vi "Get Decimal Places.vi"(8 "error in (no error)":errorcluster, 10 "Channel":T2, 11 "EPU452 in":refnum<class "EPU452.lvclass">) -> (0 "error out":errorcluster, 1 "No. of Decimal Places":T1=enum."auto", 2 "Response":string, 3 "EPU452 out":refnum<class "EPU452.lvclass">)   [LabVIEW 2018, in "EPU452.lvclass"]
uses:
  EPU452.lvclass
  Controls/Channels.ctl
  Controls/Decimal Places.ctl
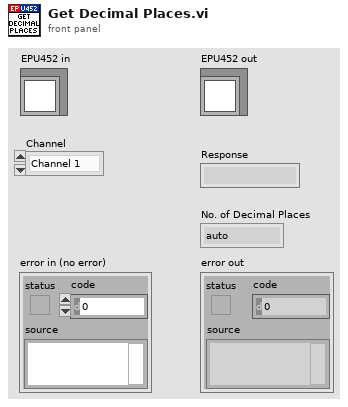
[diagram p1: front panel]
types:
  T1 = typedef "EPU452.lvclass/Decimal Places.ctl" = enum16{"0", "1", "2", "3", "4", "5", "6", "auto"}
  T2 = typedef "EPU452.lvclass/Channels.ctl" = enum16{"Channel 1", "Channel 2", "Channel 3", "Channel 4"}
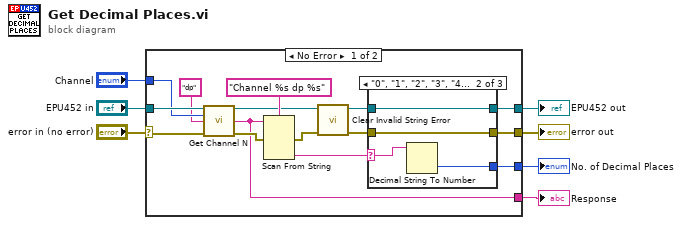
[diagram p0: block diagram]
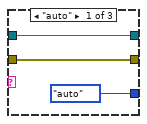
[diagram p2: hidden frame]
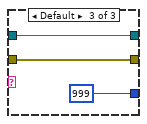
[diagram p3: hidden frame]
diagram:
  n1 = case shown="No Error" "error in (no error)" {
    selector: "error in (no error)" -> [w19 w34]
    tunnel: [w11 w34] -> w6
    tunnel: [w12 w33] -> w4
    tunnel: "EPU452 in" -> [w22 w33]
    tunnel: "Channel" -> [w21 _]
    tunnel: [w10 _] -> w2
    tunnel: [w9 _] -> w1
    frame No Error {
      n2 = call "Get Channel N.vi"("EPU452 in"=w22, "Channel"=w21, "Function"="dp", "error in (no error)"=w19) -> ("EPU452 out"=w16:refnum<class "EPU452.lvclass">, "Response"=w9:string, "error out"=w17:errorcluster)  [unwired: 9 in]
      n3 = Scan From String(format string="Channel %s dp %s" ("Function"), input string=w9, error in=w17) -> (error out=w15:errorcluster, output 2=w8:string)  [unwired: 4 in, 2 out]
      n4 = call "Clear Invalid String Error.vi"("error in (no error)"=w15, "EPU452 in"=w16) -> ("error out"=w14:errorcluster, "EPU452 out"=w13:refnum<class "EPU452.lvclass">)  [unwired: 8 in]
      n5 = case shown="\"0\", \"1\", \"2\", \"3\", \"4\", \"5\", \"6\"" w8 {
        selector: w8 -> [_ w29 _]
        tunnel: w14 -> [w24 w27 w30]
        tunnel: w13 -> [w23 w26 w31]
        tunnel: [Decimal_Places."auto" ("No. of Decimal Places") w28 999] -> w10
        tunnel: [w24 w27 w30] -> w11
        tunnel: [w23 w26 w31] -> w12
        frame "auto" {
        }
        frame "0", "1", "2", "3", "4", "5", "6" {
          n6 = Decimal String To Number(string=w29) -> (number=w28:i32)  [unwired: 2 in, 1 out]
        }
        frame Default {
        }
      }
    }
    frame Error {
    }
  }
  "error out" <- w6
  "EPU452 out" <- w4
  "No. of Decimal Places" <- w2
  "Response" <- w1
